vi "Pos ctrl window-Settings window.vi"() -> (3 "Cancelled?":bool)   [LabVIEW 2020]
doc: "Use this template to create a dialog box with event handling."
uses:
  Globals/Pos ctrl window globals.vi
  Global Variables/General Globals.vi
  Typedefs/Save-Load enum.ctl
panel:
  in  "Minimum allowed speed (um/sec)":i32=1000 min=1 max=10000 step=1
  in  "Maximum allowed speed (um/sec)":i32=100 min=1 max=50000 step=1
  in  "Speed setting increment (um/sec)":i32=1 min=1
  in  "Z Limit (+-um)":sgl=150.0 min=1 max=1000 step=1
  in  "OK":bool
  # "XYZ Movement Settings"
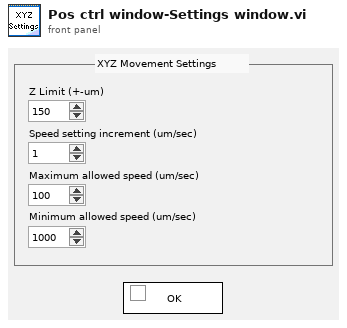
[diagram p1: front panel]
types:
  T1 = typedef "Save-Load enum.ctl" = enum16{"Save to file", "Load from file", "Compare from file", "Save Backup"}
  T2 = enum32{"Invalid", "Standard", "Closed", "Hidden", "Minimized", "Maximized"}
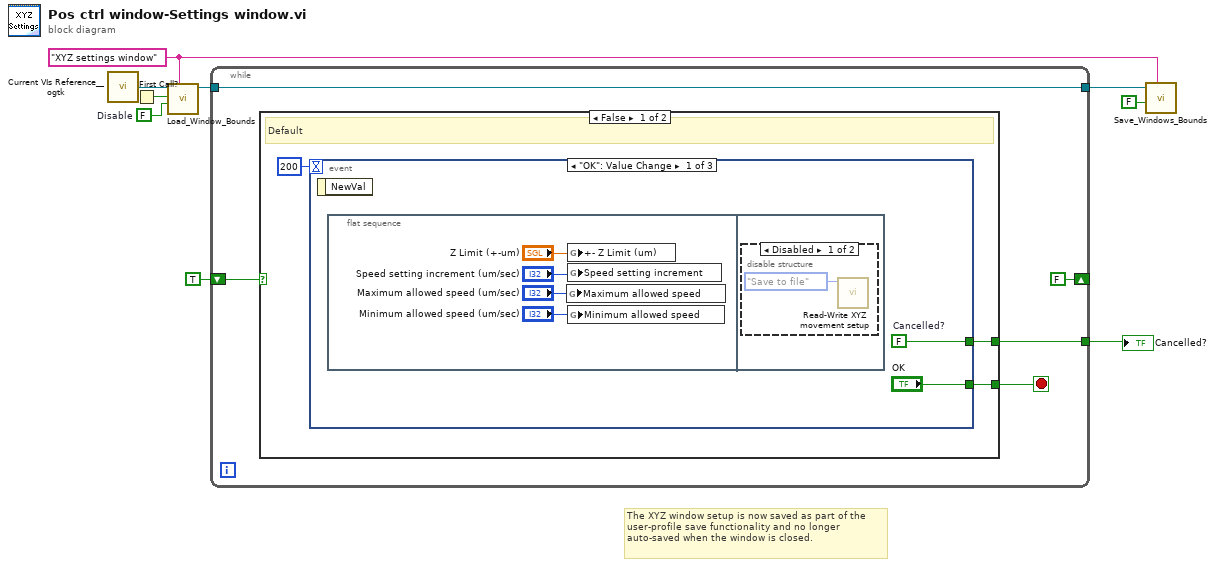
[diagram p0: block diagram]
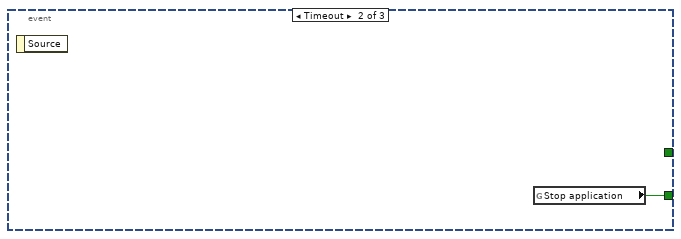
[diagram p3: hidden frame]
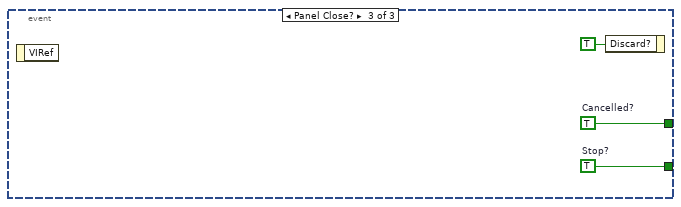
[diagram p4: hidden frame]
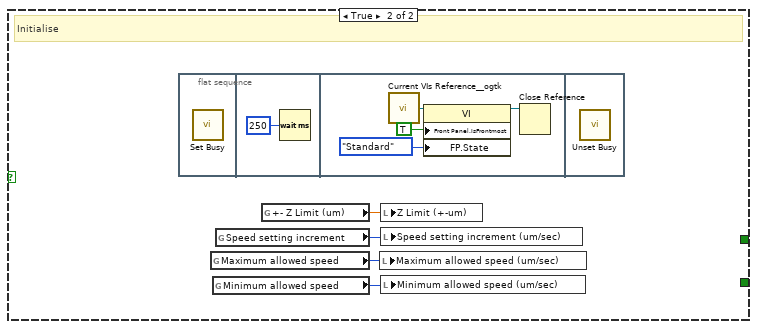
[diagram p5: hidden frame]
diagram:
  w5 = FALSE  # Disable
  w4 = "XYZ settings window" ("Window Name (i.e. Key)")
  # "The XYZ window setup is now saved as part of the user-profile save functionality and no longer auto-saved when the window is closed."
  n1 = call <userlib>:"Current VIs Reference__ogtk.vi"() -> ("Current VI's reference"=w7:refnum<vi>)  [unwired: 5 in]
  n2 = First Call?() -> (First Call?: T/F=w6:bool)
  n3 = call "Load_Window_Bounds.vi"("Window Name (i.e. Key)"=w4, "Disable"=w5, "First Call"=w6, "Window VI's Ref"=w7) -> ("reference out"=w2:refnum<vi>)  [unwired: 4 in, 3 out]
  n4 = while {
    tunnel: [w13] -> w9
    shift-right: [FALSE] -> _
    shift-left: TRUE -> [w12]
    tunnel: w2 -> [w10]
    tunnel: [w10] -> w1
    stop <- w14 stop-if-true
    n5 = case shown="False" w12 {
      tunnel: [w17 _] -> w14
      tunnel: [w16 _] -> w13
      frame False {
        # "Default"
        n6 = event shown="[0] \"OK\": Value Change" {
          selector: _ -> [_ _ _]
          dyn-events: _ -> [_ _ _]
          timeout: 200 -> [_ _ _]
          tunnel: ["OK" w25 w27] -> w17
          tunnel: [w19 _ w26] -> w16
          event "OK": Value Change {
            w19 = FALSE  # Cancelled?
            n7 = event-data() -> ()  [unwired: 1 in, 1 out]
            n8 = flat-sequence {
              frame #0 {
                n9 = global write "Pos ctrl window globals.vi" "Maximum allowed speed"("Maximum allowed speed (um/sec)") -> ()
                n10 = global write "Pos ctrl window globals.vi" "+- Z Limit (um)"("Z Limit (+-um)") -> ()
                n11 = global write "Pos ctrl window globals.vi" "Speed setting increment"("Speed setting increment (um/sec)") -> ()
                n12 = global write "Pos ctrl window globals.vi" "Minimum allowed speed"("Minimum allowed speed (um/sec)") -> ()
              }
              frame #1 {
                n13 = disable-structure shown="Disabled" {
                  frame Disabled {
                    n14 = call "Read-Write XYZ movement setup.vi"("Function"=Save-Load_enum."Save to file") -> ()  [unwired: 10 in, 1 out]
                  }
                  frame Enabled {
                  }
                }
              }
            }
          }
          event Timeout {
            n15 = event-data() -> ()  [unwired: 1 in, 1 out]
            n16 = global read "General Globals.vi" "Stop application"() -> (w25:bool)
          }
          event Panel Close? {
            w26 = TRUE  # Cancelled?
            w27 = TRUE  # Stop?
            n17 = event-data() -> ()  [unwired: 1 in, 1 out]
            n18 = event-data("Discard?"=TRUE) -> ()  [unwired: 1 in, 1 out]
          }
        }
      }
      frame True {
        # "Initialise"
        n19 = flat-sequence {
          frame #0 {
            n20 = call <vilib>:"Set Busy.vi"() -> ()  [unwired: 10 in, 2 out]
          }
          frame #1 {
            n21 = Wait (ms)(milliseconds to wait=u32 250) -> ()  [unwired: 1 out]
          }
          frame #2 {
            n22 = call <userlib>:"Current VIs Reference__ogtk.vi"() -> ("Current VI's reference"=w37:refnum<vi>)  [unwired: 5 in]
            n23 = property class="VI"(reference=w37, "Front Panel.IsFrontmost"=TRUE ("Front Panel Window:Is Frontmost"), "FP.State"=T2."Standard" ("Front Panel Window:State")) -> (reference out=w36:refnum<vi>)  [unwired: 1 in, 1 out]
            n24 = Close Reference(reference=w36) -> ()  [unwired: 1 in, 1 out]
          }
          frame #3 {
            n25 = call <vilib>:"Unset Busy.vi"() -> ()  [unwired: 11 in, 1 out]
          }
        }
        n26 = global read "Pos ctrl window globals.vi" "Maximum allowed speed"() -> (w30:i32)
        n27 = global read "Pos ctrl window globals.vi" "Minimum allowed speed"() -> (w29:i32)
        n28 = global read "Pos ctrl window globals.vi" "Speed setting increment"() -> (w31:i32)
        n29 = global read "Pos ctrl window globals.vi" "+- Z Limit (um)"() -> (w32:sgl)
        n30 = local write "Maximum allowed speed (um/sec)"(w30) -> ()
        n31 = local write "Z Limit (+-um)"(w32) -> ()
        n32 = local write "Speed setting increment (um/sec)"(w31) -> ()
        n33 = local write "Minimum allowed speed (um/sec)"(w29) -> ()
      }
    }
  }
  "Cancelled?" <- w9
  n34 = call "Save_Windows_Bounds.vi"("Window Name (i.e. Key)"=w4, "Front Panel Window:Open"=FALSE, "Window VI's Ref"=w1) -> ()  [unwired: 8 in, 1 out]
